vi "M9003ReadPhotons.vi"(9 "Prealocaed Data":u32[](array[numeric]), 10 "Number of Photons":u32, 11 "HANDLE":i32) -> (0 "Photons/Second":dbl[unit] format="%#_13g", 1 "Time":dbl[unit] format="%#_13g", 2 "Total Pulses":u32, 3 "Results":u32[](array[numeric]))   [LabVIEW 2009]
uses:
  M9003api.dll
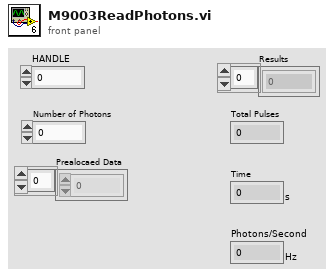
[diagram p1: front panel]
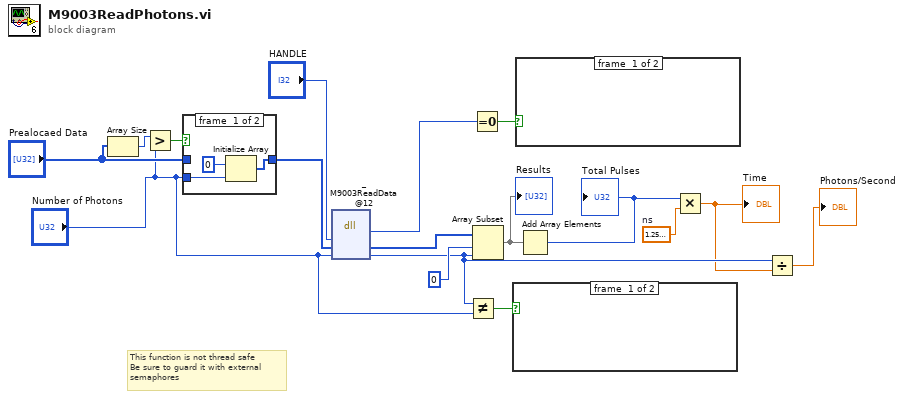
[diagram p0: block diagram]
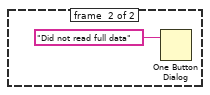
[diagram p2: hidden frame]
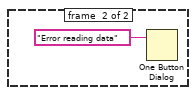
[diagram p3: hidden frame]
diagram:
  w6 = dbl[unit] 1.2500000000000001e-08  # ns
  # "This function is not thread safe\nBe sure to guard it with external\nsemaphores"
  n1 = Array Size(array="Prealocaed Data") -> (size(s)=w2:i32)
  n2 = Greater?(x=w2, y="Number of Photons") -> (0:w17:bool)
  n3 = case shown="False" w17 {
    tunnel: "Prealocaed Data" -> [_ w21]
    tunnel: [w18 w21] -> w15
    tunnel: "Number of Photons" -> [w19 _]
    frame #0 {
      n4 = Initialize Array(u32 0, w19) -> (w18:u32[])
    }
    frame #1 {
    }
  }
  n5 = dll-call lib="C:/Documents and Settings/qoptics/Desktop/Mover_2009/Sub_Vis/M9003Commands/M9003api.dll" fn="_M9003ReadData@12" label="M9003ReadData"("Handle"="HANDLE", "DataBuffer"=w15, "DataLength"="Number of Photons") -> ("return type"=w13:i32, "DataBuffer"=w10:u32[], "DataLength"=w5:u32)  [unwired: 4 in, 2 out]
  n6 = Not Equal?(x=w5, y="Number of Photons") -> (x != y?=w9:bool)
  n7 = Equal To 0?(x=w13) -> (x = 0?=w12:bool)
  n8 = Array Subset(array=w10, index=0, length=w5) -> (w8:u32[])
  "Results" <- w8
  n9 = case shown="True" w9 {
    frame #0 {
    }
    frame #1 {
      n10 = One Button Dialog(message="Did not read full data") -> ()  [unwired: 1 in, 1 out]
    }
  }
  n11 = case shown="True" w12 {
    frame #0 {
    }
    frame #1 {
      n12 = One Button Dialog(message="Error reading data") -> ()  [unwired: 1 in, 1 out]
    }
  }
  n13 = Add Array Elements(numeric array=w8) -> (sum=w7:u32)
  "Total Pulses" <- w7
  n14 = Multiply(x=w7, y=w6) -> (x*y=w4:dbl[unit])
  "Time" <- w4
  n15 = Divide(x=w5, y=w4) -> (x/y=→"Photons/Second":dbl[unit])
